vi "Actor Core.vi"(8 "error in":errorcluster, 11 "StoreUI in":refnum<class "StoreUI.lvclass">) -> (0 "error out":errorcluster, 3 "Actor out":refnum<class "Actor.lvclass">)   [LabVIEW 2015, in "StoreUI.lvlib" / "StoreUI.lvclass"]
doc: "(<B>Filename</B>: Actor Framework.lvlib:Actor.lvclass:Actor Core.vi)\n\nReceives messages to the actor, reacts to them, and initiates any error handling that may shut the actor down.\n\nDescendant classes may override this VI to append parallel tasks for the actor to complete while it handles messages. Overrides use the Call Parent Method node."
uses:
  StoreUI.lvclass
  <vilib>/ActorFramework/Actor/Actor.lvclass
  <userlib>/_XDesign Controls/HorizontalPicList XControl/HorizontalPicList.xctl
  <userlib>/_XDesign Controls/VerticalPicTextList XControl/VerticalPicTextList.xctl
  Classes/Welcome Item/Welcome.lvclass
  Classes/Instrument Information/Instrument.lvclass
  Classes/Settings Item/Settings.lvclass
  StoreUI.lvclass/StoreUI.ctl
  Classes/Settings Item/Settings.lvclass/Settings.ctl
  <vilib>/ActorFramework/Actor/Actor.lvclass/Actor.ctl
  <vilib>/ActorFramework/Message Enqueuer/Message Enqueuer.lvclass/Message Enqueuer.ctl
  <vilib>/ActorFramework/Message Enqueuer/Init from Existing Queue.vi
  <vilib>/ActorFramework/Message Enqueuer/Enqueue.vi
  <vilib>/ActorFramework/Message Priority Queue/Priority Enqueue.vi
  <vilib>/ActorFramework/Stop Msg/Stop Msg.lvclass
  <vilib>/ActorFramework/Message Enqueuer/Message Enqueuer.lvclass
  VI Store/VIStore Actor/VIStore.lvclass
panel:
  in  "Categories":i32(xcontrol)
  in  "Items":i32(xcontrol)
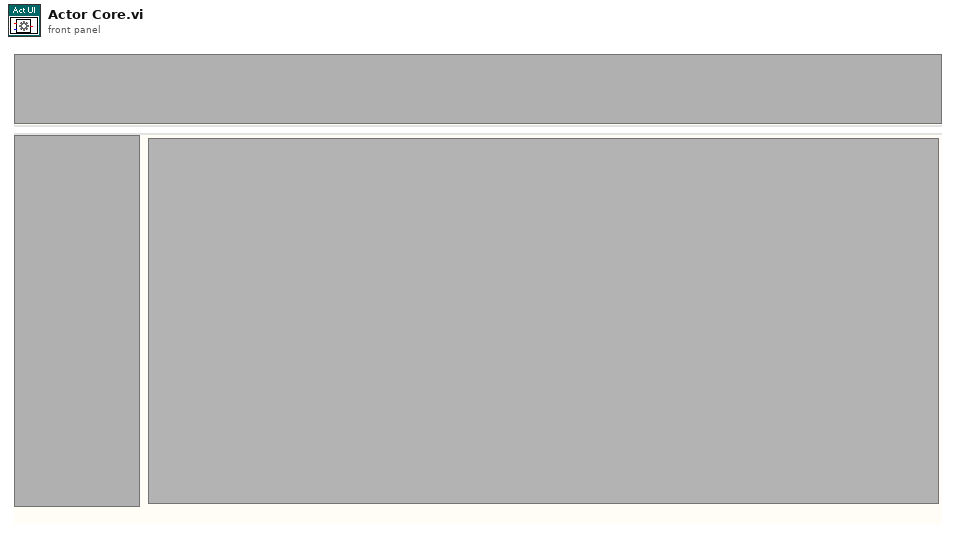
[diagram p1: front panel]
types:
  T1 = cluster{"Font Name:":string, "Size":i16, "Strikeout?":bool, "Italic?":bool, "Underline?":bool, "Outline?":bool, "Shadow?":bool, "Bold?":bool}
  T2 = typedef "imagedata.ctl" = cluster{"image type":i32, "image depth":i32, "image":u8[], "mask":u8[], "colors":u32[], "Rectangle":cluster{"left":i16, "top":i16, "right":i16, "bottom":i16}}
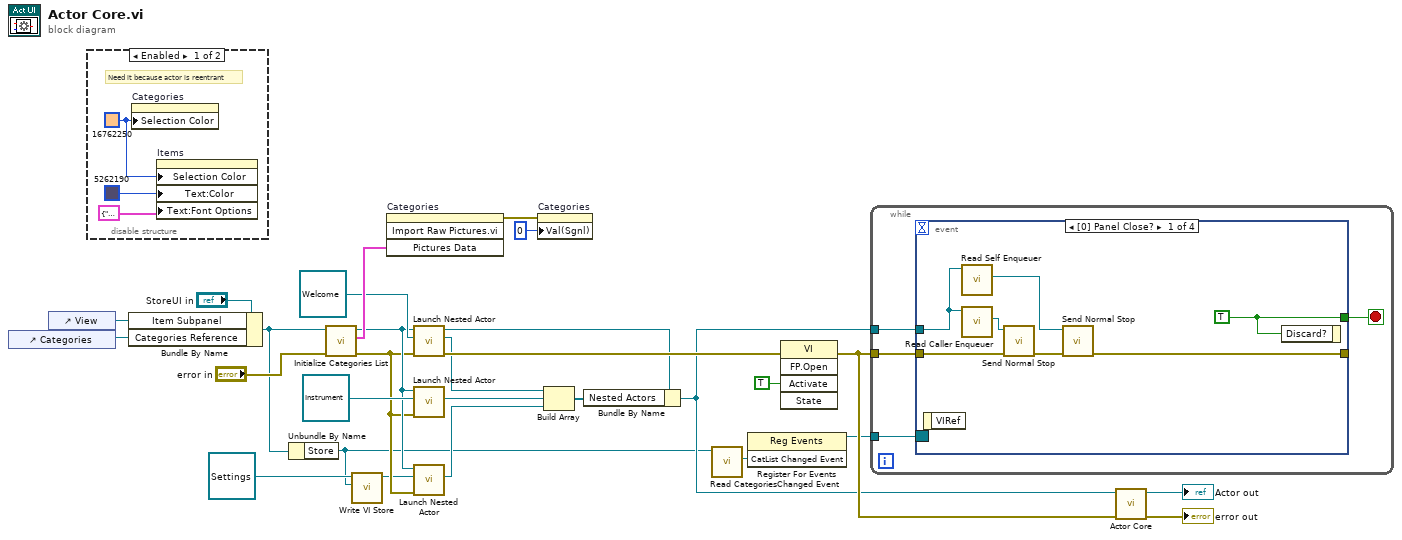
[diagram p0: block diagram]
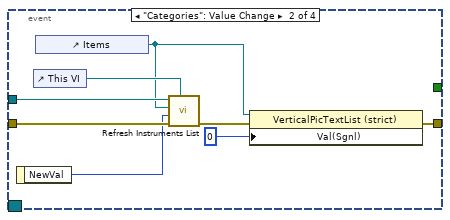
[diagram p3: hidden frame]
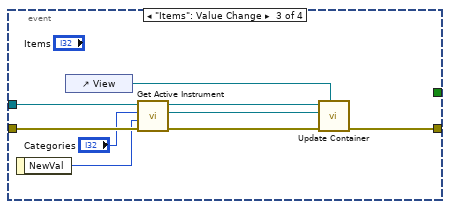
[diagram p4: hidden frame]
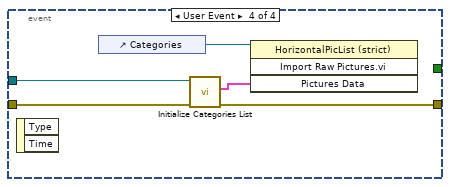
[diagram p5: hidden frame]
diagram:
  n1 = control-ref of="Categories"() -> (w16:refnum<vi>)
  n2 = control-ref of="View"() -> (w17:refnum<vi>)
  n3 = disable-structure shown="Enabled" {
    frame Enabled {
      w31 = u32 16762250
      # "Need it because actor is reentrant"
      n4 = property on="Categories" class="HorizontalPicList (strict)"("Selection Color"=w31) -> ()  [unwired: 2 in, 2 out]
      n5 = property on="Items" class="VerticalPicTextList (strict)"("Selection Color"=w31, "Text:Color"=u32 5262190, "Text:Font Options"=T1 {"Font Name:"="Euphemia", "Size"=18, "Strikeout?"=FALSE, "Italic?"=FALSE, "Underline?"=FALSE, "Outline?"=FALSE, "Shadow?"=FALSE, "Bold?"=TRUE}) -> ()  [unwired: 2 in, 2 out]
    }
    frame Disabled {
    }
  }
  n6 = Bundle By Name(cluster="StoreUI in", "Item Subpanel"=w17, "Categories Reference"=w16) -> (w5:refnum<class "StoreUI.lvclass">)
  n7 = Unbundle By Name(w5) -> ("Store"=w2:refnum<class "VIStore.lvclass">)
  n8 = call "Initialize Categories List.vi"("error in (no error)"="error in", "StoreUI in"=w5) -> ("error out"=w7:errorcluster, "Icons"=w23:T2[], "StoreUI out"=w8:refnum<class "StoreUI.lvclass">)  [unwired: 7 in]
  n9 = call "Write VI Store.vi"("VI App Store.lvlib:VIStore.lvclass"=w2, "Settings in"=refnum<class "Settings.lvclass"> refnum ("Settings.lvclass")) -> ("Settings out"=w3:refnum<class "Settings.lvclass">)  [unwired: 8 in, 1 out]
  n10 = invoke on="Categories" class="HorizontalPicList (strict)" method="Import Raw Pictures.vi"("Pictures Data"=w23) -> (error out=w22:errorcluster)  [unwired: 3 in, 3 out]
  n11 = call <vilib>:"Launch Nested Actor.vi"("error in (no error)"=w7, "Nested Actor"=refnum<class "Welcome.lvclass"> refnum ("Welcome.lvclass"), "Caller Actor in"=w8) -> ("error out"=w19:errorcluster, "Nested Actor's Enqueuer"=w11:refnum<class "Message Enqueuer.lvclass">, "Caller Actor out"=w13:refnum<class "StoreUI.lvclass">)  [unwired: 6 in]
  n12 = call <vilib>:"Launch Nested Actor.vi"("error in (no error)"=w7, "Nested Actor"=refnum<class "Instrument.lvclass"> refnum ("Instrument.lvclass"), "Caller Actor in"=w8) -> ("Nested Actor's Enqueuer"=w10:refnum<class "Message Enqueuer.lvclass">)  [unwired: 6 in, 2 out]
  n13 = call <vilib>:"Launch Nested Actor.vi"("error in (no error)"=w7, "Nested Actor"=w3, "Caller Actor in"=w8) -> ("Nested Actor's Enqueuer"=w6:refnum<class "Message Enqueuer.lvclass">)  [unwired: 6 in, 2 out]
  n14 = property on="Categories" class="HorizontalPicList (strict)"(error in=w22, "Val(Sgnl)"=0 ("Value (Signaling)")) -> ()  [unwired: 1 in, 2 out]
  n15 = Build Array(w11, w10, w6) -> (w9:refnum<class "Message Enqueuer.lvclass">[])
  n16 = Bundle By Name(cluster=w13, "Nested Actors"=w9) -> (w12:refnum<class "StoreUI.lvclass">)
  n17 = call "Read CategoriesChanged Event.vi"("VIStore in"=w2) -> ("CatList Changed Event"=w1:refnum<user-event>)  [unwired: 8 in, 2 out]
  n18 = register-events(w1) -> (reference out=w20:refnum<event-registration>)  [unwired: 2 in, 1 out]
  n19 = invoke class="VI" method="FP.Open"(error in=w19, "Activate"=TRUE ("Activate?")) -> (error out=w21:errorcluster)  [unwired: 3 in, 4 out]
  n20 = while {
    tunnel: w21 -> [w33]
    tunnel: w12 -> [w34]
    tunnel: w20 -> [w32]
    stop <- w35 stop-if-true
    n21 = event shown="[0] Panel Close?" {
      selector: w32 -> [_ _ _ _]
      dyn-events: _ -> [_ _ _ _]
      timeout: _ -> [_ _ _ _]
      tunnel: [w39 _ _ _] -> w35
      tunnel: w34 -> [w37 w49 w59 w62]
      tunnel: w33 -> [w40 w50 w58 w61]
      tunnel: [w38 w44 w56 w60] -> _
      event Panel Close? {
        w39 = TRUE ("Discard?")
        n22 = event-data() -> ()  [unwired: 1 in, 1 out]
        n23 = call <vilib>:"Read Self Enqueuer.vi"("Actor"=w37) -> ("Self Enqueuer"=w36:refnum<class "Message Enqueuer.lvclass">)  [unwired: 10 in]
        n24 = call <vilib>:"Read Caller Enqueuer.vi"("Actor"=w37) -> ("Caller Enqueuer"=w42:refnum<class "Message Enqueuer.lvclass">)  [unwired: 10 in]
        n25 = call <vilib>:"Send Normal Stop.vi"("error in (no error)"=w40, "Message Enqueuer"=w42) -> ("error out"=w41:errorcluster)  [unwired: 9 in]
        n26 = call <vilib>:"Send Normal Stop.vi"("error in (no error)"=w41, "Message Enqueuer"=w36) -> ("error out"=w38:errorcluster)  [unwired: 9 in]
        n27 = event-data("Discard?"=w39) -> ()  [unwired: 1 in, 1 out]
      }
      event "Categories": Value Change {
        n28 = event-data() -> ("NewVal"=w48:i32)  [unwired: 1 in]
        n29 = control-ref of="This VI"() -> (w47:refnum<vi>)
        n30 = control-ref of="Items"() -> (w43:refnum<vi>)
        n31 = call "Refresh Instruments List.vi"("UI Ref"=w47, "error in (no error)"=w50, "NewVal"=w48, "VerticalPicTextList Refnum"=w43, "StoreUI in"=w49) -> ("error out"=w46:errorcluster)  [unwired: 5 in, 1 out]
        n32 = property class="VerticalPicTextList (strict)"(reference=w43, error in=w46, "Val(Sgnl)"=0 ("Value (Signaling)")) -> (error out=w44:errorcluster)  [unwired: 1 out]
      }
      event "Items": Value Change {
        n33 = event-data() -> ("NewVal"=w55:i32)  [unwired: 1 in]
        n34 = control-ref of="View"() -> (w53:refnum<vi>)
        n35 = call "Get Active Instrument.vi"("error in (no error)"=w58, "Instrument Index"=w55, "Category Index"="Categories", "StoreUI in"=w59) -> ("error out"=w57:errorcluster, "Item"=w51:refnum<class "Generic Item.lvclass">, "StoreUI out"=w54:refnum<class "StoreUI.lvclass">)  [unwired: 5 in]
        n36 = call "Update Container.vi"("Container"=w53, "error in (no error)"=w57, "Item"=w51, "StoreUI"=w54) -> ("error out"=w56:errorcluster)  [unwired: 6 in, 1 out]
      }
      event User Event {
        n37 = event-data() -> ()  [unwired: 1 in, 2 out]
        n38 = control-ref of="Categories"() -> (w64:refnum<vi>)
        n39 = call "Initialize Categories List.vi"("error in (no error)"=w61, "StoreUI in"=w62) -> ("error out"=w60:errorcluster, "Icons"=w63:T2[])  [unwired: 7 in, 1 out]
        n40 = invoke class="HorizontalPicList (strict)" method="Import Raw Pictures.vi"(reference=w64, "Pictures Data"=w63) -> ()  [unwired: 2 in, 4 out]
      }
    }
  }
  n41 = call-parent "Actor Core.vi"("error in"=w21, "Actor in"=w12) -> ("error out"=→"error out":errorcluster, "Actor out"=→"Actor out":refnum<class "Actor.lvclass">)  [unwired: 8 in]
